vi "Example data inverse post-processing (single point).vi"(0 "Calibration data":T1={"X cal.[]"=[0.18323830295620053, 0.5022759108677167, 0.5926494582411277, 0.6661572393359195, 0.7738522670991032, 0.8056162976693839, 0.8978854253288069, 0.9131465104685323, 0.998198602505461, 1.0026536354542668, 1.0697031684682123, 1.0921294784978217, 1.12634848007751], "Re cal.[]"=[0.05836901900647489, 0.22234941748039563, 0.3015014894413766, 0.37907259878050203, 0.5315212662031547, 0.5843186336351215, 0.7493379557739939, 0.7811312845686427, 0.9579100635301298, 0.968544779466997, 1.1278235480081842, 1.1845542549316277, 1.2707750850078616], "a1[]"=[0.5139845410306613, 0.694908421100499, 0.9655549133380104, 1.2354182702612118, 1.5388668488196042, 1.7253155968767342, 1.935875310920986, 2.080885331144939, 2.2328002605238204, 2.3813313947618693, 2.452594226248764, 2.5246632991683033], "a2[]"=[-0.567092642319511, 3.0111150428522957, -0.009461861177446703, 2.2004140825264833, 5.776179850523374, -0.22907956125341525, 19.477407826803766, -1.871103511573675, 70.58084557623488, -1.3220160025433672, 7.094218596447346, -0.2914365144530001], "a3[]"=[1.7775103256064757, -11.166529475918521, 16.733581628717324, -4.900141213800908, -59.63298736273686, 9.899216022714324, -643.3109334585097, 21.66651332028892, -8067.401298929666, 18.428518110921583, -163.1245085960374, 4.25840177969994]}, 5 "U (m/s)":dbl=3.97034, 7 "Ta (°C)":dbl=20.4382, 9 "Overheat ratio (Rw / R0)":dbl=1.7, 11 "Gain":dbl=10.0, 12 "Offset (V)":dbl=0.512) -> (4 "V_out (V)":dbl=2.077060256143217)   [LabVIEW 2022 SP3]
doc: "Example VI for how to inverse post-process recorded flow speed values to obtain the associated bridge voltage, point-by-point.\nPN 15-OCT-24."
uses:
  Ctls/Calibration data.ctl
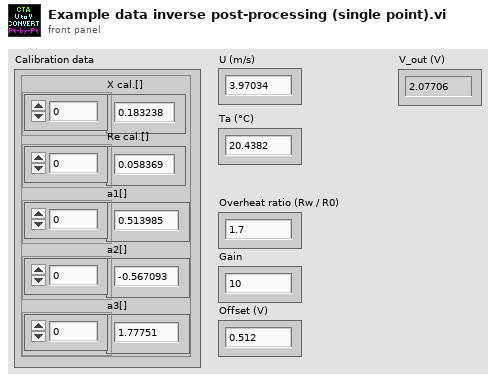
[diagram p1: front panel]
types:
  T1 = typedef "Calibration data.ctl" = cluster{"X cal.[]":dbl[], "Re cal.[]":dbl[], "a1[]":dbl[], "a2[]":dbl[], "a3[]":dbl[]}
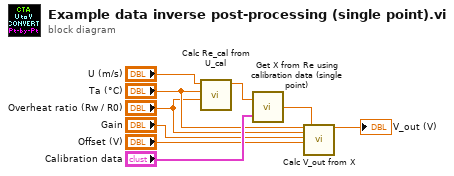
[diagram p0: block diagram]
diagram:
  n1 = call "Calc Re_cal from U_cal.vi"("Overheat ratio (Rw / R0)"="Overheat ratio (Rw / R0)", "Ta (°C)"="Ta (°C)", "U_cal (m/s)"="U (m/s)") -> ("Re"=w1:dbl)  [unwired: 8 in]
  n2 = call "Get X from Re using calibration data (single point).vi"("Calibration data"="Calibration data", "Re"=w1) -> ("X"=w5:dbl)
  n3 = call "Calc V_out from X.vi"("Ta (°C)"="Ta (°C)", "Overheat ratio (Rw / R0)"="Overheat ratio (Rw / R0)", "Gain"="Gain", "Offset (V)"="Offset (V)", "X"=w5) -> ("V_out (V)"=→"V_out (V)":dbl)  [unwired: 14 in]
